vi "CNV Graph.vi"() -> ()   [LabVIEW 2016]
panel:
  out "Boolean":bool
  out "Waveform Graph":i32[][](graph)
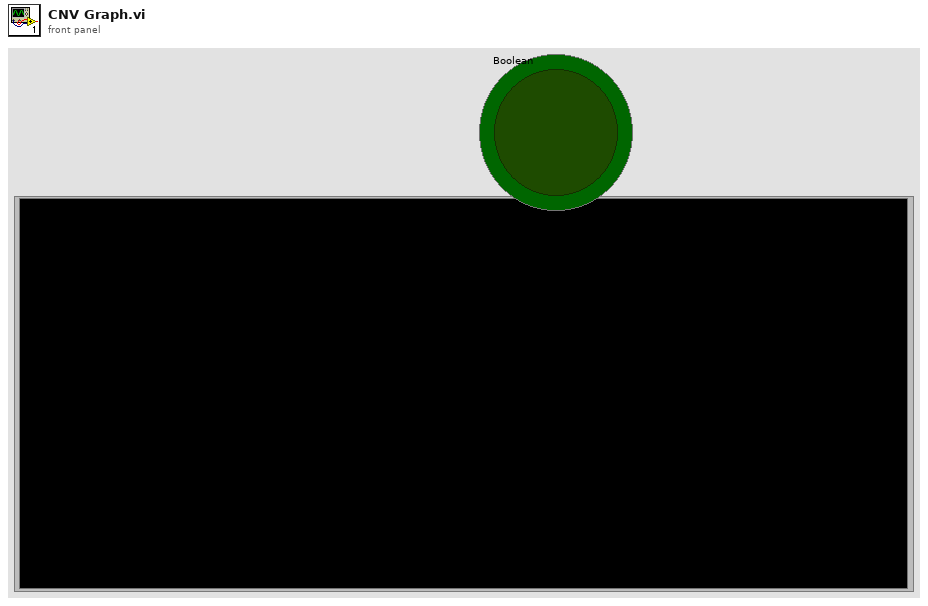
[diagram p1: front panel]
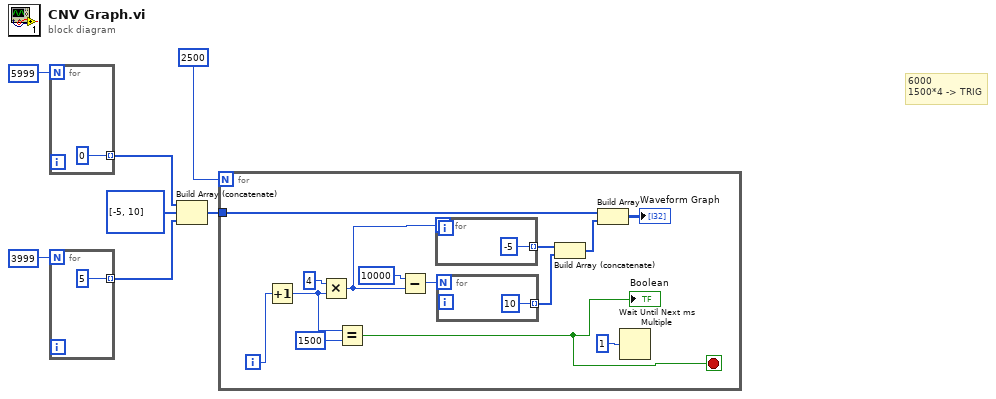
[diagram p0: block diagram]
diagram:
  # "6000\n1500*4 -> TRIG"
  n1 = for {
    N: 5999 -> [_]
    tunnel: [0] -> w3 mode=indexing
  }
  n2 = for {
    N: 3999 -> [_]
    tunnel: [5] -> w5 mode=indexing
  }
  n3 = Build Array (concatenate)(w3, i32[] [-5, 10], w5) -> (w1:i32[])
  n4 = for {
    N: 2500 -> [_]
    tunnel: w1 -> [w13]
    i -> [w19]
    stop <- w10 stop-if-true
    n5 = Increment(x=w19) -> (x+1=w12:i32)
    n6 = Multiply(x=4, y=w12) -> (x*y=w15:i32)
    n7 = Equal?(x=w12, y=1500) -> (x = y?=w10:bool)
    "Boolean" <- w10
    n8 = Subtract(x=10000, y=w15) -> (x-y=w17:i32)
    n9 = for {
      N: w15 -> [_]
      tunnel: [-5] -> w21 mode=indexing
    }
    n10 = for {
      N: w17 -> [_]
      tunnel: [10] -> w22 mode=indexing
    }
    n11 = Build Array (concatenate)(w21, w22) -> (w20:i32[])
    n12 = Build Array(w13, w20) -> (→"Waveform Graph":i32[][])
    n13 = Wait Until Next ms Multiple(millisecond multiple=u32 1) -> ()  [unwired: 1 out]
  }
